vi "PH_Sequencer.destructor.vi"(0 "i ref in":refnum<vi>, 5 "error in(no error)":errorcluster) -> (19 "error out":errorcluster)   [LabVIEW 2014, in "PH_Sequencer.lvlib"]
doc: "This is the destructor of a class.\n\nLicense Agreement for this software:\n\nCopyright (C)\nGesellschaft für Schwerionenforschung, GSI\nPlanckstr. 1\n64291 Darmstadt\nGermany\n\nContact: D.Beck@gsi.de \n\nThis program is free software; you can redistribute it and/or modify it under the terms of the \nGNU General Public License as published by the Free Software Foundation; either version 2 of \nthe license, or (at your option) any later version.\n\nThis program is distributed in the hope that it will be useful, but WITHOUT ANY WARRANTY; \nwithout even the implied warranty of MERCHANTABILITY or FITNESS FOR A PARTICULAR PURPOSE. See the GNU General License for more details (http://www.gnu.org).\n\nGesellschaft für Schwerionenforschung, GSI\nPlanckstr. 1, 64291 Darmstadt, Germany\nFor all questions and ideas contact: M.Richter@gsi.de, H.Brand@gsi.de or D.Beck@gsi.de.\nLast update: 16-JUN-2004"
uses:
  PH_Sequencer.lvlib
  PH_Classes/PH_Calorimeter_USB/PH_Calorimeter_USB.lvlib
  CSlibraries-extern/DimLVEvent/LVDimInterface/LVDimInterface.lvlib
  PH_Devices/PH_TKTDS-30xx/PH_TKTDS-30xx.lvlib
  PH_BL-Master/PH_BL-Master.lvlib
  PH_BeamlineController/PH_BeamlineController.lvlib
  PH_Basics/PH_PSDBWriter/PH_PSDBWriter.lvlib
  PH_Basics/PH_SM_Class/PH_SM_Class.lvlib
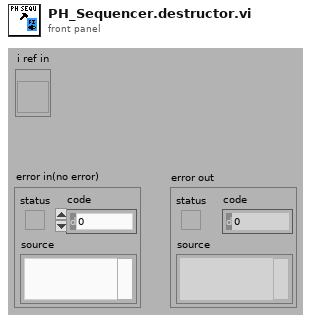
[diagram p1: front panel]
types:
  T1 = typedef "PH_Sequencer.lvlib/PH_Sequencer.i attribute.ctl" = cluster{"GUI Refs":cluster{"Main Off":refnum<vi>, "Fire":refnum<vi>, "Status":refnum<vi>, "Ready":refnum<vi>, "Waiting Time":refnum<vi>, "Timeout":refnum<vi>, "PPMA Ready":refnum<vi>, "Sequencer SM State":refnum<vi>, "PPPA Ready":refnum<vi>, "Calorimeter":refnum<vi>, "Beamline Ready":refnum<vi>, "Clear Beamline":refnum<vi>, "Linkage PPMA Rods":refnum<vi>, "Linkage Current PA":refnum<vi>, "Linkage Current MA":refnum<vi>, "Timing Ready":refnum<vi>, "State Timing":refnum<vi>, "Force Timing":refnum<vi>, "PSDB Shot Comment":refnum<vi>, "State PA Backreflection":refnum<vi>, "Beamline Z6 Ready":refnum<vi>, "Clear Z6 Beamline":refnum<vi>, "Sequence length":refnum<vi>, "Timing Mode":refnum<vi>, "Slow Trigger Settings":refnum<vi>, "Experiment Description":refnum<vi>, "State PSDB":refnum<vi>, "PSDB Ready":refnum<vi>, "Set PSDB Settings":refnum<vi>, "Get PSDB Info":refnum<vi>, "Take Snapshot":refnum<vi>, "Shottype":refnum<vi>, "Experiment":refnum<vi>, "Phase Frontends":refnum<vi>, "PP 45mm PILC in use":refnum<vi>}, "Status Info":cluster{"Machine Status":T2, "WaitingTime":i32, "Timeout":bool}, "Readyness":cluster{"Ready to shot":bool, "PPMA Ready":bool, "PPPA Ready":bool, "BL Ready":bool, "Timing Ready":bool, "BL Z6 Ready":bool, "PSDBReady":bool}, "Instancenames":cluster{"PPMA Rods":string, "PP Current Meas":string, "PH Beamline Chief":string, "PA Backrefl Meas":string, "Z6 Beamline Chief":string}, "Data to read":bool, "Calorimeter":cluster{"Instancename":string, "On":bool, "linked":bool}, "Linkage":cluster{"PPMA Rods":bool, "PP Current Meas":bool, "PHELIX Beamline Chief":bool, "PA Backrefl Meas":bool, "Z6 Beamline Chief":bool}, "Timing":cluster{"Instance":string, "linked":bool, "Status":T2, "Timing Mode":T3, "Slow Trigger Settings":T4, "Info available":cluster{"ext SlowTrigger":bool, "T2":bool, "Mode":bool, "Delay Slow Trigger":bool, "Phase FEs":bool}, "FE Phase":T5}, "Service ID R2S":i32, "PSDB":cluster{"Controller Instance":string, "Controller Status":T2, "Controller linked":bool, "Settings acknowledged":bool, "Current Experiment ID":i16, "Current Shot Type":i16, "Current Comment":string, "Remember Settings":bool, "Write 2 early":bool}, "PSDB Data":cluster{"Main Off?":bool, "Sequence Length":dbl, "Sequence startet":timestamp}, "6P 4Q Positions":cluster{"Instancename":string, "linked":bool, "Position":T6}[], "PUs":T7[]}
  T2 = typedef "PH_StatusHandler.lvlib/PH_StatusHandler.Status.ctl" = i16
  T3 = typedef "PH_Timing.lvlib/PH_Timing.Timing Mode.ctl" = cluster{"T2":i16, "Modeselector":enum32{"10 Hz", "0.5 Hz", "Shot"}}
  T4 = typedef "PH_Timing.lvlib/PH_Timing.Slow Trigger Settings.ctl" = cluster{"Delay":dbl, "externally triggered?":bool}
  T5 = typedef "PH_Timing.lvlib/PH_Timing.Phase FEs.ctl" = cluster{"Phase":dbl}
  T6 = typedef "PH_4_Pos_Selector.lvlib/PH_4_Pos_Selector.Position Selector.ctl" = u16
  T7 = typedef "PH_Sequencer.lvlib/PH_Sequencer.Head.ctl" = cluster{"PowerUnit":T8, "GUI Ref":refnum<vi>, "Information":T9, "linked?":bool, "GUI Ref Current Voltage":refnum<vi>}
  T8 = typedef "PH_PP_Common.lvlib/PH_PP_Common.PUs.ctl" = enum16{"no Info", "PA-19mm-1", "PA-19mm-2", "PA-45mm-PILC", "PA-45mm-MAIN", "MA-PU-1", "MA-PU-2", "MA-PU-3", "MA-PU-4", "MA-PU-5", "MA-PU-6", "MA-FR", "MA-PILC", "PA-45mm-DP"}
  T9 = typedef "PH_Sequencer.lvlib/PH_Sequencer.PU Information.ctl" = cluster{"State":T2, "Waiting Time [s]":dbl, "PU State SM":T10, "PU Timeout SM":T10}
  T10 = typedef "PH_PowerUnit_BaseClass.lvlib/PH_PowerUnit_BaseClass.SM States.ctl" = enum16{".", "Stand by", "Switch PU on", "Configure", "Set Default Voltage", "Set STANDBY", "Set READY", "Wait for Shot Cmd", "Open Dump Rods", "Open Ross Relais", "Close Ross Relais", "Switch PSU on", "Switch PSU off", "Charge", "Switch GD Channel on", "Close Dump Rods", "Rods-TO", "RR-TO", "PSU-TO", "Trigger-TO"}
  T11 = enum16{"SetAttribute", "GetAttribute", "CreateAttribute", "DestroyAttribute", "DestroyAllAtributes"}
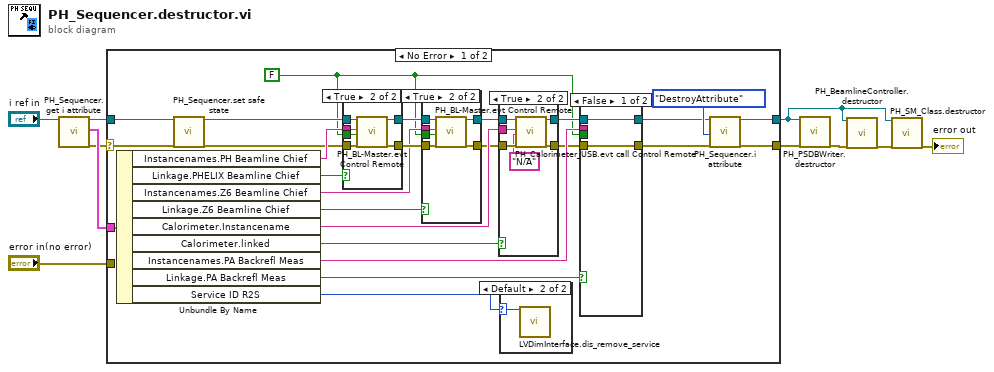
[diagram p0: block diagram]
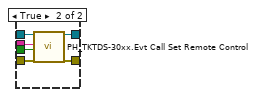
[diagram p4: hidden frame]
diagram:
  n1 = call "PH_Sequencer.get i attribute.vi"("i ref in"="i ref in") -> ("i ref out"=w9:refnum<vi>, "i attribute"=w10:T1, "error out"=w7:errorcluster)  [unwired: 16 in]
  n2 = case shown="No Error" w7 {
    selector: w7 -> [w14 _]
    tunnel: w10 -> [w35 _]
    tunnel: [w21 w71] -> w3
    tunnel: [w20 w70] -> w1
    tunnel: w9 -> [w18 w70]
    tunnel: "error in(no error)" -> [_ w71]
    frame No Error {
      w11 = FALSE
      n3 = Unbundle By Name(w35) -> ("Instancenames.PH Beamline Chief"=w34:string, "Linkage.PHELIX Beamline Chief"=w33:bool, "Instancenames.Z6 Beamline Chief"=w26:string, "Linkage.Z6 Beamline Chief"=w25:bool, "Calorimeter.Instancename"=w32:string, "Calorimeter.linked"=w31:bool, "Instancenames.PA Backrefl Meas"=w30:string, "Linkage.PA Backrefl Meas"=w29:bool, "Service ID R2S"=w24:i32)
      n4 = call "PH_Sequencer.set safe state.vi"("i ref in"=w18, "error in (no error)"=w14) -> ("i ref out"=w17:refnum<vi>, "error out"=w19:errorcluster)  [unwired: 16 in]
      n5 = case shown="True" w33 {
        tunnel: w17 -> [w63 w69]
        tunnel: w19 -> [w62 w68]
        tunnel: w34 -> [_ w67]
        tunnel: w11 -> [_ w66]
        tunnel: [w63 w65] -> w27
        tunnel: [w62 w64] -> w28
        frame False {
        }
        frame True {
          n6 = call "PH_BL-Master.evt Control Remote.vi"("i ref in"=w69, "Instance"=w67, "Control Remote"=w66, "error in (no error)"=w68) -> ("i ref out"=w65:refnum<vi>, "error out"=w64:errorcluster)  [unwired: 14 in]
        }
      }
      n7 = case shown="True" w25 {
        tunnel: w27 -> [w39 w45]
        tunnel: w28 -> [w38 w44]
        tunnel: w26 -> [_ w43]
        tunnel: w11 -> [_ w42]
        tunnel: [w39 w41] -> w23
        tunnel: [w38 w40] -> w22
        frame False {
        }
        frame True {
          n8 = call "PH_BL-Master.evt Control Remote.vi"("i ref in"=w45, "Instance"=w43, "Control Remote"=w42, "error in (no error)"=w44) -> ("i ref out"=w41:refnum<vi>, "error out"=w40:errorcluster)  [unwired: 14 in]
        }
      }
      n9 = case shown="True" w31 {
        tunnel: w23 -> [w54 w61]
        tunnel: [w54 w60] -> w16
        tunnel: w22 -> [w55 w59]
        tunnel: [w55 w58] -> w15
        tunnel: w32 -> [_ w57]
        frame False {
        }
        frame True {
          n10 = call "PH_Calorimeter_USB.evt call Control Remote.vi"("i ref in"=w61, "Instance"=w57, "Owner"="N/A", "error in (no error)"=w59) -> ("i ref out"=w60:refnum<vi>, "error out"=w58:errorcluster)  [unwired: 14 in]
        }
      }
      n11 = case shown="Default" w24 {
        selector: w24 -> [_ w37]
        frame -1 {
        }
        frame Default {
          n12 = call "LVDimInterface.dis_remove_service.vi"("my_serviceID"=w37) -> ()  [unwired: 18 in, 1 out]
        }
      }
      n13 = case shown="False" w29 {
        tunnel: w30 -> [_ w53]
        tunnel: w15 -> [w46 w52]
        tunnel: [w46 w51] -> w13
        tunnel: w16 -> [w47 w50]
        tunnel: [w47 w49] -> w12
        tunnel: w11 -> [_ w48]
        frame False {
        }
        frame True {
          n14 = call "PH_TKTDS-30xx.Evt Call Set Remote Control.vi"("i ref in"=w50, "Instance"=w53, "Ctrl Remote?"=w48, "error in (no error)"=w52) -> ("i ref out"=w49:refnum<vi>, "error out"=w51:errorcluster)  [unwired: 14 in]
        }
      }
      n15 = call "PH_Sequencer.i attribute.vi"("VI Refnum"=w12, "Action"=T11."DestroyAttribute", "error in (no error)"=w13) -> ("VI Refnum out"=w20:refnum<vi>, "error out"=w21:errorcluster)  [unwired: 14 in, 1 out]
    }
    frame Error {
    }
  }
  n16 = call "PH_PSDBWriter.destructor.vi"("i ref in"=w1, "error in(no error)"=w3) -> ("error out"=w5:errorcluster)  [unwired: 17 in]
  n17 = call "PH_BeamlineController.destructor.vi"("i ref in"=w1, "error in(no error)"=w5) -> ("error out"=w4:errorcluster)  [unwired: 17 in]
  n18 = call "PH_SM_Class.destructor.vi"("i ref in"=w1, "error in(no error)"=w4) -> ("error out"=→"error out":errorcluster)  [unwired: 17 in]
